vi "set_soft_limits.vi"(8 "error in (no error)":errorcluster caption="错误输入（无错误）", 10 "soft limits":cluster{"min":dbl, "max":dbl}[](array[cluster]), 11 "MotorSystem输入":refnum<class "MotorSystem.lvclass">) -> (0 "error out":errorcluster caption="错误输出", 3 "MotorSystem输出":refnum<class "MotorSystem.lvclass">)   [LabVIEW 2016, in "MotionControl_UFO_3DOF.lvlib" / "MotorSystem.lvclass"]
uses:
  <userlib>/MotionControl_UFO_3DOF/MotorSystem/MotorSystem.lvclass
  <userlib>/MotionControl_UFO_3DOF/MotorSystem/MotorSystem.lvclass/MotorSystem.ctl
  <userlib>/MotionControl_UFO_3DOF/OneMotion/OneMotion.lvclass/OneMotion.ctl
  <userlib>/MotionControl_UFO_3DOF/OneMotion/OneMotion.lvclass
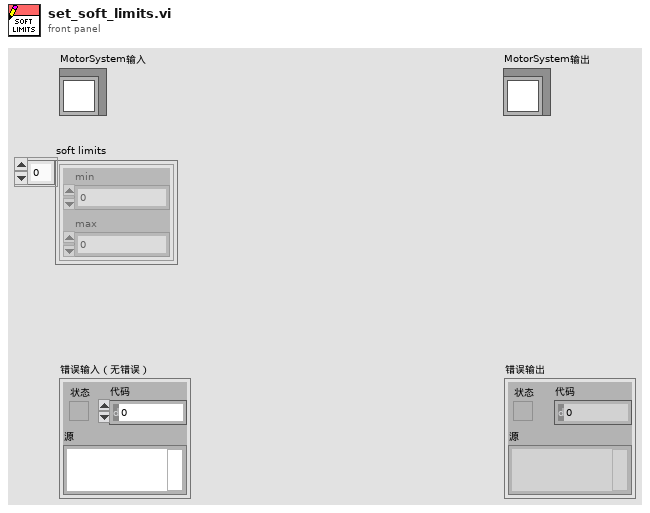
[diagram p1: front panel]
types:
  T1 = typedef "MotionControl_UFO_3DOF.lvlib/MotorSystem.lvclass/MotionCluster.ctl" = cluster{"OneMotion.lvclass":refnum<class "OneMotion.lvclass">, "connected?":bool, "default enabled?":bool, "enabled?":bool}
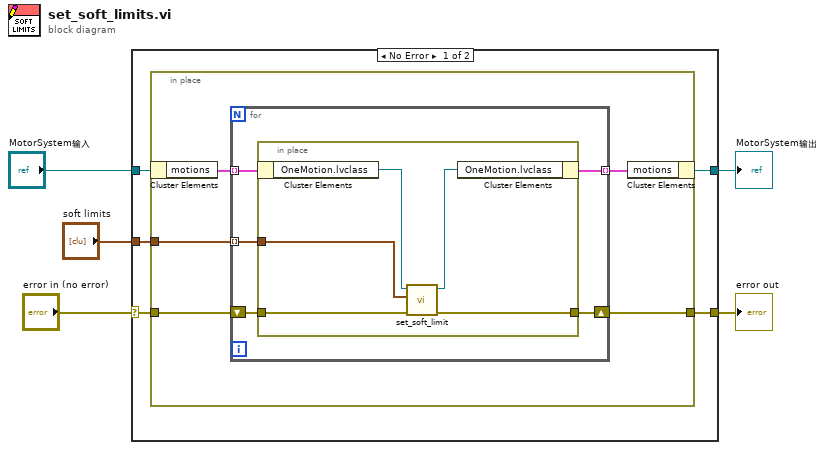
[diagram p0: block diagram]
diagram:
  n1 = case shown="No Error" "error in (no error)" {
    selector: "error in (no error)" -> [w7 w26]
    tunnel: [w6 w26] -> w4
    tunnel: [w8 w27] -> w2
    tunnel: "MotorSystem输入" -> [w10 w27]
    tunnel: "soft limits" -> [w9 _]
    frame No Error {
      n2 = in-place {
        in-place-border: w9 -> [w14]
        in-place-border: w7 -> [w12]
        in-place-border: [w11] -> w6
        n3 = in-place-cluster #1(w10) -> ("motions"=w15:T1[])
        n4 = for {
          tunnel: w15 -> [w20] mode=indexing
          tunnel: w14 -> [w19] mode=indexing
          tunnel: [w18] -> w13 mode=indexing
          shift-right: [w16] -> w11
          shift-left: w12 -> [w17]
          n5 = in-place {
            in-place-border: w19 -> [w24]
            in-place-border: w17 -> [w22]
            in-place-border: [w21] -> w16
            n6 = in-place-cluster #2(w20) -> ("OneMotion.lvclass"=w25:refnum<class "OneMotion.lvclass">)
            n7 = call <userlib>:"set_soft_limit.vi"("error in (no error)"=w22, "soft limit"=w24, "OneMotion输入"=w25) -> ("error out"=w21:errorcluster, "OneMotion输出"=w23:refnum<class "OneMotion.lvclass">)  [unwired: 7 in]
            n8 = in-place-cluster #2("OneMotion.lvclass"=w23) -> (w18:T1)
          }
        }
        n9 = in-place-cluster #1("motions"=w13) -> (w8:refnum<class "MotorSystem.lvclass">)
      }
    }
    frame Error {
    }
  }
  "error out" <- w4
  "MotorSystem输出" <- w2
